vi "GetTDSegLen.vi"(8 "error in":errorcluster) -> (0 "error out":errorcluster, 3 "SegLen":u8)   [LabVIEW 2012]
uses:
  bin/OVA32.dll
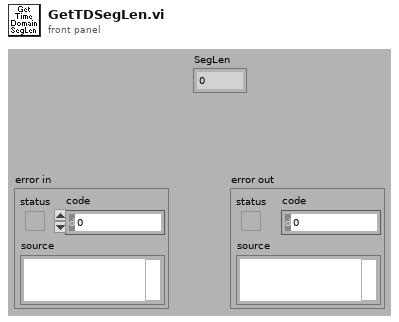
[diagram p1: front panel]
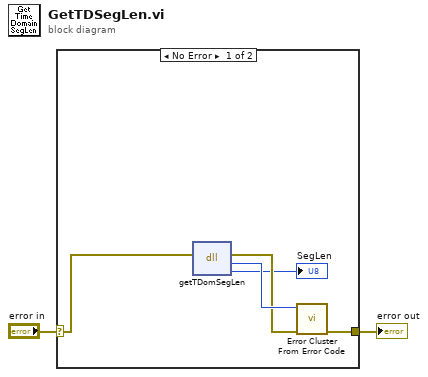
[diagram p0: block diagram]
diagram:
  n1 = case shown="No Error" "error in" {
    selector: "error in" -> [w7 w8]
    tunnel: [w4 w8] -> w1
    frame No Error {
      n2 = dll-call lib="C:/_src/OVA5000_DSP_falcon/Software/LabVIEW/OVA/SDK/OVA_5000_SDK_v5.14.3/bin/OVA32.dll" fn="getTDomSegLen"(error in=w7) -> (error out=w5:errorcluster, "return type"=w6:i32, "SegLen"=→"SegLen":u8)  [unwired: 3 in, 1 out]
      n3 = call <vilib>:"Error Cluster From Error Code.vi"("error in (no error)"=w5, "error code (0)"=w6) -> ("error out"=w4:errorcluster)  [unwired: 7 in]
    }
    frame Error {
    }
  }
  "error out" <- w1
